vi "Read Smart Relay Info DVR.vi"(8 "error in":errorcluster, 10 "DeviceID":T2, 11 "EMS Generic in":refnum<class "EMS Generic.lvclass">) -> (0 "error out":errorcluster, 2 "SmartRelay_Info":T1, 3 "EMS Generic out":refnum<class "EMS Generic.lvclass">, 4 "valid?":bool)   [LabVIEW 2018, in "EMS Generic Actor.lvlib" / "EMS Generic.lvclass"]
uses:
  EMS Generic.lvclass
  <vilib>/ORNL/CSEISMIC DDS/CSEISMIC DDS Base/Data Types/Controls/DeviceID.ctl
  <vilib>/ORNL/CSEISMIC DDS/CSEISMIC DDS Base/Data Types/SmartRelay_Info.ctl
  EMS Generic.lvclass/EMS Generic.ctl
  <vilib>/ORNL/CSEISMIC DDS/CSEISMIC DDS Base/CSEISMIC DDS.lvclass
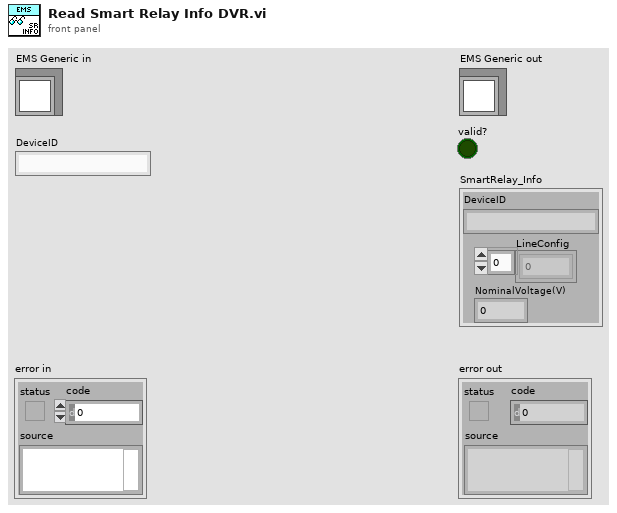
[diagram p1: front panel]
types:
  T1 = typedef "CSEISMIC DDS.lvlib/CSEISMIC DDS.lvclass/SmartRelay_Info.ctl" = cluster{"DeviceID":T2, "LineConfig":u8[], "NominalVoltage(V)":dbl}
  T2 = typedef "CSEISMIC DDS.lvlib/CSEISMIC DDS.lvclass/DeviceID.ctl" = string
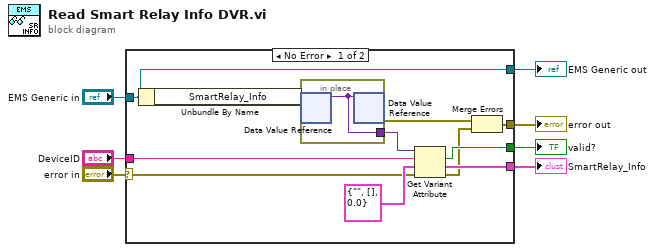
[diagram p0: block diagram]
diagram:
  n1 = case shown="No Error" "error in" {
    selector: "error in" -> [w10 w21]
    tunnel: [w16 w21] -> w6
    tunnel: [w18 w20] -> w4
    tunnel: "EMS Generic in" -> [w18 w20]
    tunnel: "DeviceID" -> [w14 _]
    tunnel: [w12 _] -> w2
    tunnel: [w11 _] -> w1
    frame No Error {
      n2 = Unbundle By Name(w18) -> ("SmartRelay_Info"=w17:refnum<data-value>)
      n3 = in-place {
        in-place-border: [w19] -> w15
        n4 = in-place-dvr #1(w17) -> (w19:variant)  [unwired: 1 out]
        n5 = in-place-dvr #1(w19) -> (w8:errorcluster)  [unwired: 1 out]
      }
      n6 = Get Variant Attribute(Variant=w15, name=w14, default value (empty Variant)=T1 {"DeviceID"="", "LineConfig"=[], "NominalVoltage(V)"=0.0} ("SmartRelay_Info"), error in=w10) -> (found=w11:bool, value=w12:T1, error out=w9:errorcluster)  [unwired: 1 out]
      n7 = Merge Errors(w8, w9) -> (w16:errorcluster)
    }
    frame Error {
    }
  }
  "error out" <- w6
  "EMS Generic out" <- w4
  "SmartRelay_Info" <- w2
  "valid?" <- w1
